vi "Parse Request.vi"(8 "error in (no error)":errorcluster, 10 "JSON Request":string, 11 "Response":refnum<class "Response.lvclass">) -> (0 "error out":errorcluster, 1 "params":variant, 2 "method":string, 3 "Response out":refnum<class "Response.lvclass">)   [LabVIEW 2016, in "Response.lvclass"]
uses:
  Response.lvclass
  typedefs/JSON-RPC-Request Object--Cluster.ctl
  Response.lvclass/Response.ctl
  <vilib>/addons/_JKI.lib/Serialization/JSON/JKI JSON Serialization.lvlib
  JSON-RPC.lvclass
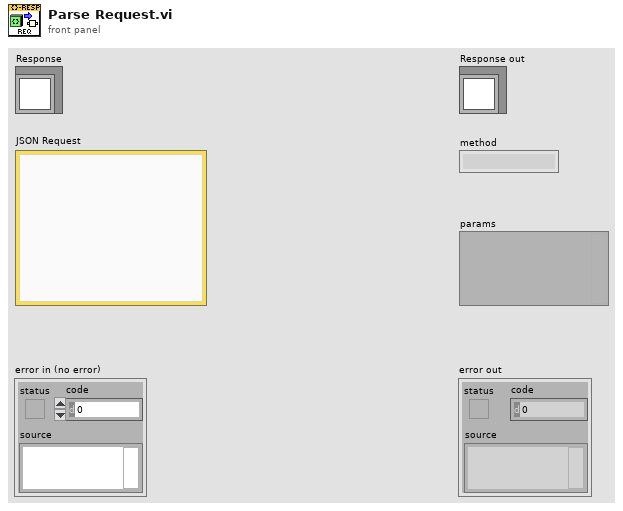
[diagram p1: front panel]
types:
  T1 = typedef "JSON-RPC.lvclass/JSON-RPC-Request Object--Cluster.ctl" = cluster{"jsonrpc":string, "method":string, "params":variant, "id":string}
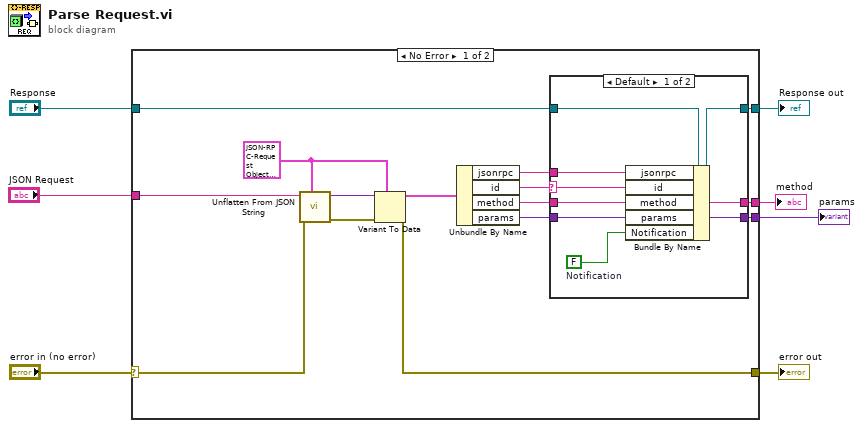
[diagram p0: block diagram]
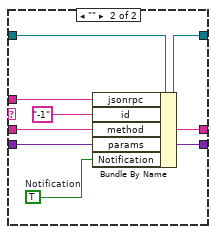
[diagram p2: hidden frame]
diagram:
  n1 = case shown="No Error" "error in (no error)" {
    selector: "error in (no error)" -> [w14 w38]
    tunnel: [w20 w38] -> w6
    tunnel: [w18 w37] -> w4
    tunnel: "Response" -> [w19 w37]
    tunnel: "JSON Request" -> [w17 _]
    tunnel: [w9 _] -> w2
    tunnel: [w8 _] -> w1
    frame No Error {
      w16 = T1 {"jsonrpc"="", "method"="", "params"=variant, "id"=""} ("Array")
      n2 = call <vilib>:"Unflatten From JSON String.vi"("Type and Defaults"=w16, "error in (no error)"=w14, "JSON String"=w17) -> ("error out"=w21:errorcluster, "Variant"=w22:variant)  [unwired: 7 in]
      n3 = Variant To Data(error in=w21, type=w16, Variant=w22) -> (data=w15:T1, error out=w20:errorcluster)
      n4 = Unbundle By Name(w15) -> ("jsonrpc"=w13:string, "id"=w11:string, "method"=w12:string, "params"=w10:variant)
      n5 = case shown="Default" w11 {
        selector: w11 -> [w29 _]
        tunnel: w19 -> [w27 w36]
        tunnel: [w26 w35] -> w18
        tunnel: w13 -> [w28 w34]
        tunnel: w12 -> [w24 w30]
        tunnel: w10 -> [w23 w31]
        tunnel: [w23 w31] -> w9
        tunnel: [w24 w30] -> w8
        frame Default {
          w25 = FALSE  # Notification
          n6 = Bundle By Name(cluster=w27, "jsonrpc"=w28, "id"=w29, "method"=w24, "params"=w23, "Notification"=w25) -> (w26:refnum<class "Response.lvclass">)
        }
        frame "" {
          w32 = TRUE  # Notification
          n7 = Bundle By Name(cluster=w36, "jsonrpc"=w34, "id"="-1", "method"=w30, "params"=w31, "Notification"=w32) -> (w35:refnum<class "Response.lvclass">)
        }
      }
    }
    frame Error {
    }
  }
  "error out" <- w6
  "Response out" <- w4
  "method" <- w1
  "params" <- w2
